vi "UDP Data Link - Driver Utilities - UDP to Rx Data.vi"(6 "Protocol Info":cluster{"ProtocolId":u8, "ProtocolRev":u8}={"ProtocolId"=1, "ProtocolRev"=8} {"ProtocolRev" format="%b"; "ProtocolId" format="%b"}, 7 "Rx Initial Values":dbl[](array[numeric]), 8 "error in (no error)":errorcluster, 10 "In4Ver":u16, 11 "UDP Data":string) -> (0 "error out":errorcluster, 1 "Error Code":i32, 3 "Rx Data":dbl[](array[numeric]))   [LabVIEW 2012, in "UDP Data Link Engine.lvlib"]
doc: "This VI converts the data received in a UDP packet into header information and Rx Channel data. It parses the header for packet size, protocol id and revision, sequence number, system definition version. and timestamp.\n\nIf the packet size, protocol id and revision or system definition does not match the expected value, the appropriate error is thrown and Rx channel data is not updated. If the sequence number does not match the most recent sequence number sent in the Tx packet, an error is thrown but Rx channel data is updated. Errors are thrown in order of importance: protocol id/rev, packet size, system definition version, sequence number.\n\nThe timestamp received in the header is used to record when the last error was received. This VI returns Rx Channel Data, Time of Last Error, Last Error Code, and Sequence Number to be written to the RT FIFO. All but the Sequence Number are updated to VeriStand channels. The sequence number is used for timeout/synchronization purposes by the inline VI."
uses:
  UDP Data Link Engine.lvlib
  <vilib>/NI Veristand/Custom Device Tools/Custom Device Utility Library/Custom Device Utility Library.lvlib
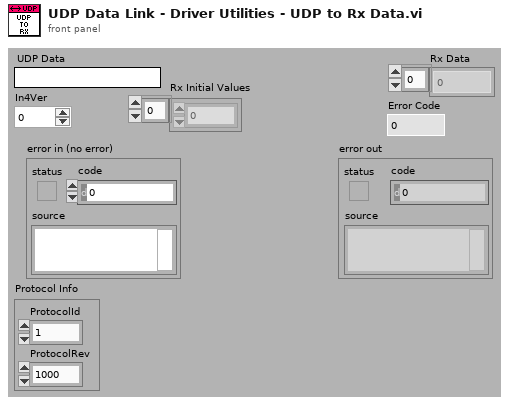
[diagram p1: front panel]
types:
  T1 = enum16{"big-endian, network order", "native, host order", "little-endian"}
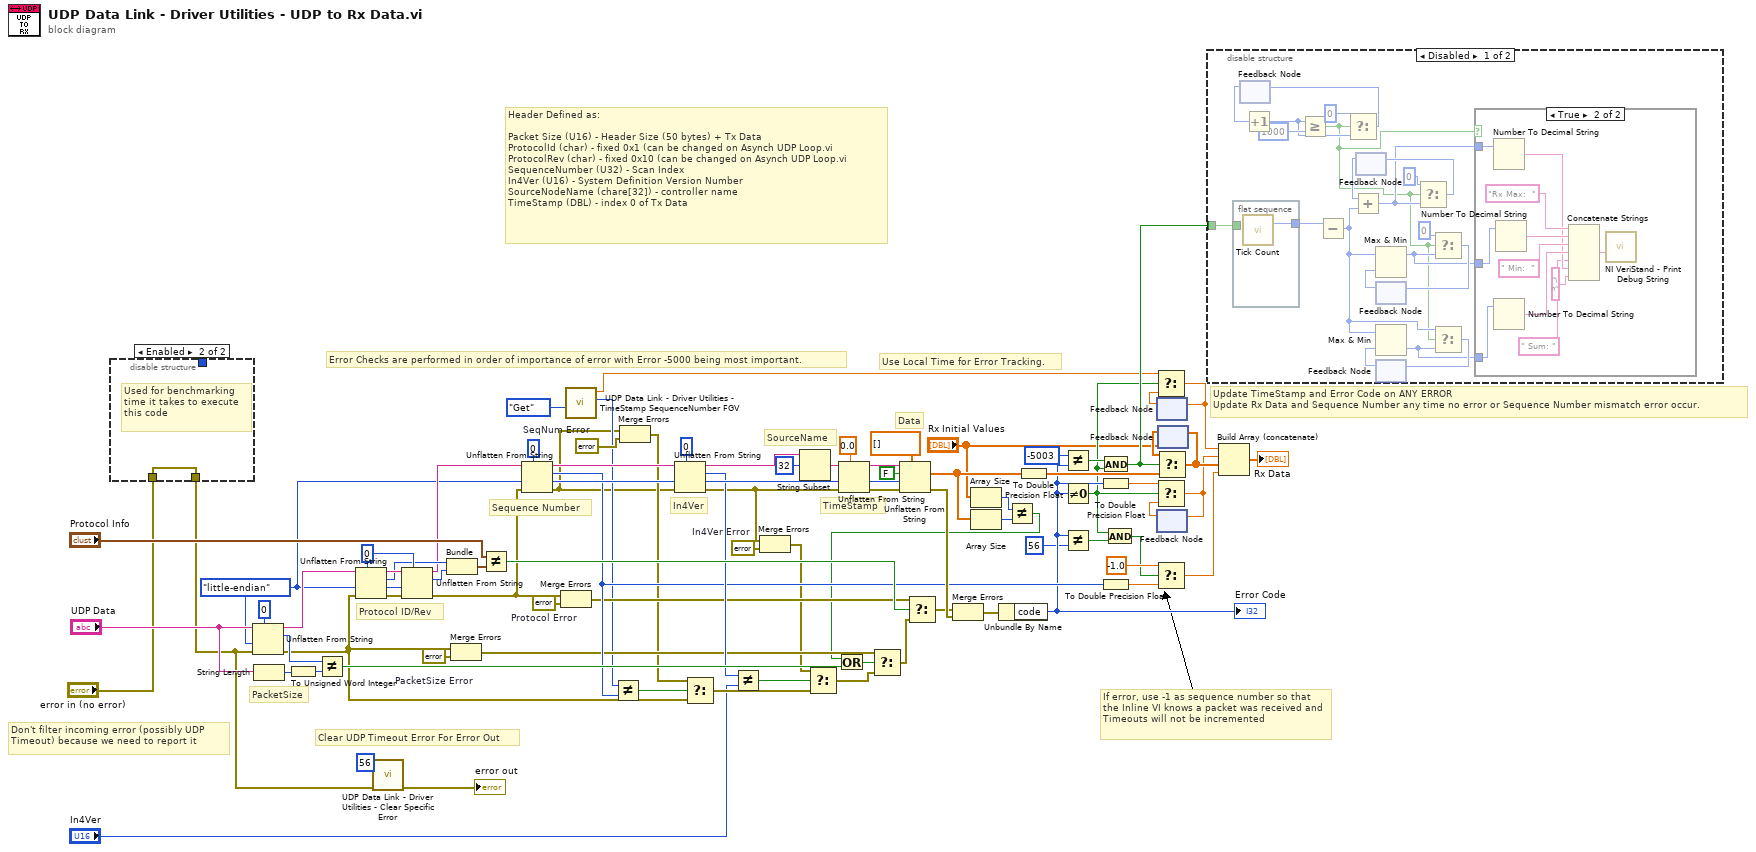
[diagram p0: block diagram]
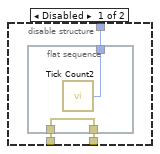
[diagram p4: hidden frame]
diagram:
  w20 = errorcluster {"status"=TRUE, "code"=-5002, "source"=""}  # In4Ver Error
  w22 = errorcluster {"status"=TRUE, "code"=-5003, "source"=""}  # SeqNum Error
  w23 = errorcluster {"status"=TRUE, "code"=-5000, "source"=""}  # Protocol Error
  w27 = errorcluster {"status"=TRUE, "code"=-5001, "source"=""}  # PacketSize Error
  w73 = u8 0
  w56 = T1."little-endian" ("byte order (0:big-endian, network order)")
  # "Use Local Time for Error Tracking."
  # "If error, use -1 as sequence number so that the Inline VI knows a packet was received and Timeouts will not be incremented"
  # "Header Defined as:\n\nPacket Size (U16) - Header Size (50 bytes) + Tx Data\nProtocolId (char) - fixed 0x1 (can be changed on Asynch UDP Loop.vi\nProtocolRev (char) - fixed 0x10 (can be changed on Asynch UDP Loop.vi\nSequenceNumber (U32) - Scan Index\nIn4Ver (U16) - System Definition Version Number\nSourceNodeName (chare[32]) - controller name\nTimeStamp (DBL) - index 0 of Tx Data"
  # "Update TimeStamp and Error Code on ANY ERROR\nUpdate Rx Data and Sequence Number any time no error or Sequence Number mismatch error occur."
  # "Don't filter incoming error (possibly UDP Timeout) because we need to report it"
  # "Data"
  # "TimeStamp"
  # "SourceName"
  # "Error Checks are performed in order of importance of error with Error -5000 being most important."
  # "In4Ver"
  # "Sequence Number"
  # "Protocol ID/Rev"
  # "PacketSize"
  # "Clear UDP Timeout Error For Error Out"
  n1 = disable-structure shown="Enabled" {
    disable-tunnel: "error in (no error)" -> [w87 w90]
    disable-tunnel: [w86 w90] -> w29
    disable-tunnel: [w85 _] -> _
    frame Disabled {
      n2 = flat-sequence {
        tunnel: w87 -> [w89]
        tunnel: [w89] -> w86
        tunnel: [w88] -> w85
        frame #0 {
          n3 = call "Tick Count2"() -> ("Tick Count(uSec)"=w88:u32)
        }
      }
    }
    frame Enabled {
      # "Used for benchmarking time it takes to execute this code"
    }
  }
  n4 = Unflatten From String(type=u16 0, binary string="UDP Data", byte order (0:big-endian, network order)=w56, error in (no error)=w29) -> (rest of the binary string=w76:string, value=w60:u16, error out=w28:errorcluster)  [unwired: 1 in]
  n5 = String Length(string="UDP Data") -> (length=w77:i32)
  n6 = To Unsigned Word Integer(number=w77) -> (unsigned 16bit integer=w61:u16)
  n7 = Not Equal?(x=w60, y=w61) -> (x != y?=w78:bool)
  n8 = Unflatten From String(type=w73, binary string=w76, byte order (0:big-endian, network order)=w56, error in (no error)=w28) -> (rest of the binary string=w74:string, value=w71:u8, error out=w75:errorcluster)  [unwired: 1 in]
  n9 = call "UDP Data Link - Driver Utilities - Clear Specific Error.vi"("Error to Clear"=56, "Error In"=w29) -> ("Error Out"=→"error out":errorcluster)  [unwired: 6 in, 1 out]
  n10 = Unflatten From String(type=w73, binary string=w74, byte order (0:big-endian, network order)=w56, error in (no error)=w75) -> (rest of the binary string=w59:string, value=w72:u8, error out=w25:errorcluster)  [unwired: 1 in]
  n11 = Bundle(w71, w72) -> (w69:cluster{u8, u8})  [unwired: 1 in]
  n12 = Merge Errors(w28, w27) -> (w26:errorcluster)
  n13 = Not Equal?(x="Protocol Info", y=w69) -> (x != y?=w70:bool)
  n14 = Unflatten From String(type=u32 0, binary string=w59, byte order (0:big-endian, network order)=w56, error in (no error)=w25) -> (rest of the binary string=w57:string, value=w35:u32, error out=w7:errorcluster)  [unwired: 1 in]
  n15 = Merge Errors(w25, w23) -> (w24:errorcluster)
  n16 = call "UDP Data Link - Driver Utilities - TimeStamp SequenceNumber FGV.vi"("Enum"=enum16{"Get", "Set"}."Get") -> ("Sequence Number Out"=w16:u32, "Timestamp Out"=w9:dbl)  [unwired: 8 in, 1 out]
  n17 = Not Equal?(x=w16, y=w35) -> (x != y?=w41:bool)
  n18 = Merge Errors(w7, w22) -> (w21:errorcluster)
  n19 = Unflatten From String(type=u16 0, binary string=w57, byte order (0:big-endian, network order)=w56, error in (no error)=w7) -> (rest of the binary string=w50:string, value=w38:u16, error out=w19:errorcluster)  [unwired: 1 in]
  n20 = Select(t=w21, s=w41, f=w28) -> (s? t:f=w54:errorcluster)
  n21 = Not Equal?(x=w38, y="In4Ver") -> (x != y?=w52:bool)
  n22 = Merge Errors(w19, w20) -> (w18:errorcluster)
  n23 = String Subset(string=w50, offset (0)=32) -> (substring=w49:string)  [unwired: 1 in]
  n24 = Select(t=w18, s=w52, f=w54) -> (s? t:f=w53:errorcluster)
  n25 = Unflatten From String(type=0.0, binary string=w49, byte order (0:big-endian, network order)=w56, error in (no error)=w19) -> (rest of the binary string=w65:string, error out=w67:errorcluster)  [unwired: 1 in, 1 out]
  n26 = Unflatten From String(type=sgl[] [], binary string=w65, data includes array or string size? (T)=FALSE, byte order (0:big-endian, network order)=w56, error in (no error)=w67) -> (value=w5:sgl[], error out=w63:errorcluster)  [unwired: 1 out]
  n27 = Array Size(array="Rx Initial Values") -> (size(s)=w3:i32)
  n28 = Array Size(array=w5) -> (size(s)=w6:i32)
  n29 = Not Equal?(x=w3, y=w6) -> (x != y?=w1:bool)
  n30 = Or(x=w1, y=w78) -> (x .or. y?=w2:bool)
  n31 = Select(t=w26, s=w2, f=w53) -> (s? t:f=w62:errorcluster)
  n32 = Select(t=w24, s=w70, f=w62) -> (s? t:f=w51:errorcluster)
  n33 = Merge Errors(w51, w63) -> (w44:errorcluster)
  n34 = Unbundle By Name(w44) -> ("code"=w13:i32)
  "Error Code" <- w13
  n35 = To Double Precision Float(number=w5) -> (double precision float=w46:dbl[])
  n36 = Not Equal?(x=-5003 ("error code (0)"), y=w13) -> (x != y?=w40:bool)
  n37 = Not Equal To 0?(x=w13) -> (x != 0?=w10:bool)
  n38 = Not Equal?(x=w13, y=56 ("Error to Clear")) -> (x != y?=w14:bool)
  n39 = And(x=w40, y=w10) -> (x .and. y?=w31:bool)
  n40 = To Double Precision Float(number=w13) -> (double precision float=w34:dbl)
  n41 = To Double Precision Float(number=w35) -> (double precision float=w33:dbl)
  n42 = And(x=w10, y=w14) -> (x .and. y?=w11:bool)
  n43 = Select(t=-1.0, s=w11, f=w33) -> (s? t:f=w32:dbl)
  n44 = feedback #1() -> (w80:dbl)  [unwired: 1 in]
  n45 = Select(t=w9, s=w10, f=w80) -> (s? t:f=w8:dbl)
  n46 = feedback-in #1(w8) -> ()
  n47 = feedback #2() -> (w81:dbl)  [unwired: 1 in]
  n48 = Select(t=w34, s=w10, f=w81) -> (s? t:f=w36:dbl)
  n49 = feedback-in #2(w36) -> ()
  n50 = feedback #3("Rx Initial Values") -> (w45:dbl[])
  n51 = Select(t=w45, s=w31, f=w46) -> (s? t:f=w42:dbl[])
  n52 = feedback-in #3(w42) -> ()
  n53 = disable-structure shown="Disabled" {
    disable-tunnel: w31 -> [w110 _]
    frame Disabled {
      n54 = flat-sequence {
        tunnel: w110 -> [_]
        tunnel: [w111] -> w109
        frame #0 {
          n55 = call "Tick Count"() -> ("Tick Count(uSec)"=w111:u32)
        }
      }
      n56 = feedback #4() -> (w108:i32)  [unwired: 1 in]
      n57 = Increment(x=w108) -> (x+1=w104:i32)
      n58 = Greater Or Equal?(x=w104, y=1000) -> (x >= y?=w91:bool)
      n59 = Subtract(x=w109) -> (x-y=w98:u32)  [unwired: 1 in]
      n60 = Select(t=0, s=w91, f=w104) -> (s? t:f=w106:i32)
      n61 = feedback-in #4(w106) -> ()
      n62 = feedback #5() -> (w103:u32)  [unwired: 1 in]
      n63 = Add(x=w103, y=w98) -> (x+y=w92:u32)
      n64 = feedback #6() -> (w101:u32)  [unwired: 1 in]
      n65 = Max & Min(x=w98, y=w101) -> (max(x,y)=w93:u32)  [unwired: 1 out]
      n66 = feedback #7() -> (w99:u32)  [unwired: 1 in]
      n67 = Max & Min(x=w98, y=w99) -> (min(x,y)=w94:u32)  [unwired: 1 out]
      n68 = Select(t=u32 0, s=w91, f=w92) -> (s? t:f=w95:u32)
      n69 = feedback-in #5(w95) -> ()
      n70 = Select(t=u32 0, s=w91, f=w93) -> (s? t:f=w97:u32)
      n71 = feedback-in #6(w97) -> ()
      n72 = Select(t=w98, s=w91, f=w94) -> (s? t:f=w96:u32)
      n73 = feedback-in #7(w96) -> ()
      n74 = case shown="True" w91 {
        tunnel: w94 -> [_ w115]
        tunnel: w93 -> [_ w114]
        tunnel: w92 -> [_ w113]
        frame False {
        }
        frame True {
          n75 = Number To Decimal String(number=w113) -> (decimal integer string=w117:string)  [unwired: 1 in]
          n76 = Number To Decimal String(number=w115) -> (decimal integer string=w119:string)  [unwired: 1 in]
          n77 = Number To Decimal String(number=w114) -> (decimal integer string=w122:string)  [unwired: 1 in]
          n78 = Concatenate Strings("Rx Max:  " ("string"), w122, " Min:  " ("string"), w119, " Sum: " ("string"), w117, "\n" ("string")) -> (w121:string)
          n79 = call <vilib>:"NI VeriStand - Print Debug String.vi"("Debug String"=w121) -> ()  [unwired: 9 in, 1 out]
        }
      }
    }
    frame Enabled {
      # "Used for benchmarking this code. On a 8130, it was measured to have max execution time of ~90 usec, min execution time of ~13 usec, and average execution time of ~17.7 usec. There were only 4 Rx channels being received when making this benchmark."
    }
  }
  n80 = Build Array (concatenate)(w8, w36, w42, w32) -> (→"Rx Data":dbl[])
